vi "accept.vi"(8 "error in (no error)":errorcluster, 10 "Visitor":refnum<class "Visitor.lvclass">, 11 "CompoundShape in":refnum<class "CompoundShape.lvclass">) -> (0 "error out":errorcluster, 2 "String":string, 3 "CompoundShape out":refnum<class "CompoundShape.lvclass">)   [LabVIEW 2018, in "CompoundShape.lvclass"]
uses:
  CompoundShape.lvclass
  Visitor Class/Visitor.lvclass
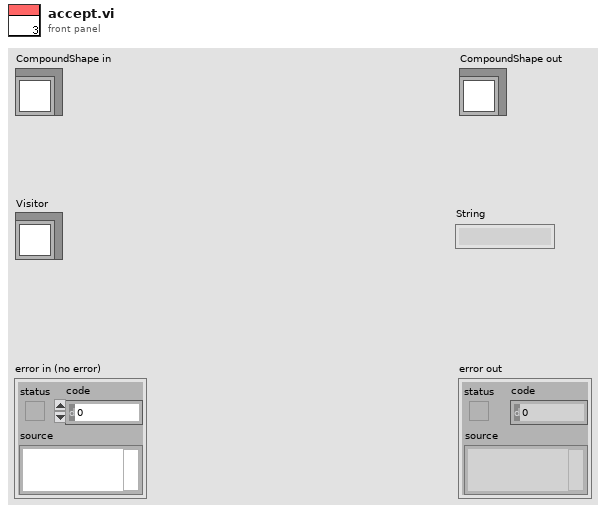
[diagram p1: front panel]
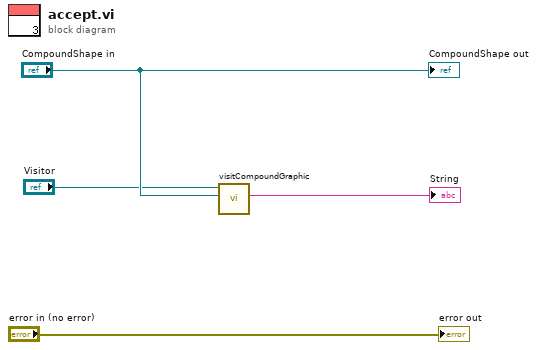
[diagram p0: block diagram]
diagram:
  n1 = call-dynamic "visitCompoundGraphic.vi"("CompoundShape"="CompoundShape in", "Visitor in"="Visitor") -> ("String"=→"String":string)  [unwired: 7 in, 2 out]
  "error out" <- "error in (no error)"
  "CompoundShape out" <- "CompoundShape in"
